vi "PathPlanner_Ctrl_LTVExecute.vi"(4 "Period":dbl=0.02, 5 "LTV_Unicycle_Ctrl_Model":T1={"Max linear ctrl effort M/S"=1.0, "Max angular ctrl effort Rad/S"=2.0, "Max Heading Meas Tol Rad"=0.2, "Max X Pos Meas Tol M"=0.0625, "Max Y Pos Meas Tol M"=0.125, "Max Linear Vel M/S"=9.0} {"Max Linear Vel M/S" format="%#_13g"; "Max Y Pos Meas Tol M" format="%#_13g"; "Max X Pos Meas Tol M" format="%#_13g"; "Max Heading Meas Tol Rad" format="%#_13g"; "Max angular ctrl effort Rad/S" format="%#_13g"; "Max linear ctrl effort M/S" format="%#_13g"}, 6 "Max Speed M/S":dbl=4.0, 7 "LTV_Unicycle_Ctrl_Tolerance":T2={"Max Heading Tolerance Rad"=1.0, "Max X Tolerance M"=2.0, "Max Y Tolerance M"=0.2} {"Max Y Tolerance M" format="%#_13g"; "Max X Tolerance M" format="%#_13g"; "Max Heading Tolerance Rad" format="%#_13g"}, 8 "Enabled":bool=TRUE, 9 "Track Width Meters":dbl=1.0, 10 "PathPlannerState":T8={"TimeSeconds"=0.0, "VelocityMPS"=0.0, "AccerationMpsSq"=0.0, "HeadingAngularVelRadPerSec"=0.0, "PositionMeters"={"X"=0.0, "Y"=0.0}, "Heading"={"VALUE"=0.0, "COS"=1.0, "SIN"=0.0}, "TargetHolonomicRotation"={"VALUE"=0.0, "COS"=1.0, "SIN"=0.0}, "CurvatureRadPerMeter"=0.0, "PathPlannerConstraints"={"MaxVelocityMps;"=0.0, "MaxAccelerationMpsSq;"=0.0, "MaxAngularVelRadPsEc;"=0.0, "MaxAngularAccRadPSecSq"=0.0, "Exists"=FALSE}, "DeltaPos"=0.0} {"TargetHolonomicRotation"."SIN" format="%13.4f"; "TargetHolonomicRotation"."COS" format="%13.4f"; "TargetHolonomicRotation"."VALUE" format="%13.4f"; "Heading"."SIN" format="%13.4f"; "Heading"."COS" format="%13.4f"; "Heading"."VALUE" format="%13.4f"; "PositionMeters"."Y" format="%14.3f"; "PositionMeters"."X" format="%14.3f"}, 11 "Current Pose SI":T4={"TRANSLATION"={"X"=0.0, "Y"=0.0}, "ROTATION"={"VALUE"=0.0, "COS"=1.0, "SIN"=0.0}} {"ROTATION"."SIN" format="%13.4f"; "ROTATION"."COS" format="%13.4f"; "ROTATION"."VALUE" format="%13.4f"; "TRANSLATION"."Y" format="%14.3f"; "TRANSLATION"."X" format="%14.3f"}) -> (0 "Position Error M":dbl, 1 "At Reference":bool, 2 "Normalized Right Wheel Dmd M/S":dbl, 3 "Normalized Left Wheel Dmd M/S":dbl)   [LabVIEW 2019, in "PathPlanner24.lvlib"]
doc: "Calculates the next output of the path following controller for differential drive robots using a LTV (linear time varying) Unicycle controller. This wraps a LTV Control function with the particulars needed to follow a PathPlanner trajectory.\n\nInputs:\n - LTV_Unicycle_Ctrl_Model - cluster - The modeling paraameters for the LTV drive controller. These are static. They should not be changed after the first call to this function.\n - UniCycle_Ctrl_Tolerance SI - pose2d - The control paraameters for the LTV drive controller. These are static. They should not be changed after the first call to this function.\n - CurrentPoseSi - pose2d - The current pose calculated by odometry or pose estimation. The pose can be absolute or relative depending on what type of trajectory is being followed.\n - PathPlannerState - cluster - The path palnner trajectory state containing the desired position and velocities of the robot.\n - TrackWidth M - doubler - The effective width of the drive track width in meters.:\n - Enabled - boolean - When TRUE, closed loop control is enabled. (Optional. Default: TRUE)\n - MaxWheelSpeed - double - The maximum speed of the drive wheels M/S.\n - Period - double - The loop period in seconds for this controller. (Optional. Default: 0.020)\n\nOutputs:\n - NormalizedLeftWheelSpeedDmd - The desired speed for the left drive wheel in SI units. The left and right speeds have been normalized so not to exceed the maximum allowed speed.\n - NormalizedRightWheelSpeedDmd - The desired speed for the right drive wheel in SI units. The left and right speeds have been normalized so not to exceed the maximum allowed speed.\n - AtReference - boolean - TRUE if the robots position is within the defined tolerance.\n - PositionError - double - Position error in SI units. How far the robot is away from the desired trajectory position."
uses:
  PathPlanner24.lvlib
  <vilib>/Rock Robotics/WPI/ThirdParty/JAS_Junk/TrajLib/TypeDef/POSE2D.ctl
  <vilib>/Rock Robotics/WPI/ThirdParty/JAS_Junk/TrajLib/TypeDef/TRANSLATION2D.ctl
  <vilib>/Rock Robotics/WPI/ThirdParty/JAS_Junk/TrajLib/TypeDef/ROTATION2D.ctl
  TypeDef/PathPlannerTrajectoryState.ctl
  TypeDef/PathPlannerPathConstraints.ctl
  <vilib>/Rock Robotics/WPI/ThirdParty/JAS_Junk/TrajLib/TypeDef/LTV_UNICYCLE_CONTROLLER.ctl
  <vilib>/Rock Robotics/WPI/ThirdParty/JAS_Junk/TrajLib/TypeDef/FUNCTION_GENERATOR_MATRIX.ctl
  <vilib>/Rock Robotics/WPI/ThirdParty/JAS_Junk/TrajLib/TypeDef/LTV_UNICYCLE_CONTROLLER_TOLERANCE.CTL
  <vilib>/Rock Robotics/WPI/ThirdParty/JAS_Junk/TrajLib/TypeDef/LTV_UNICYCLE_CONTROLLER_MODEL_PARAMS.CTL
  <vilib>/Rock Robotics/SystemInterfaces/NetworkCommunication/NetComm_UsageReport_report.vi
  <vilib>/Rock Robotics/WPI/ThirdParty/JAS_Junk/TrajLib/Pose2d_New_TRRO.vi
  <vilib>/Rock Robotics/WPI/ThirdParty/JAS_Junk/TrajLib/Util_CalcDist.vi
  <vilib>/Rock Robotics/WPI/ThirdParty/JAS_Junk/TrajLib/Globals/Util_LibraryGlobals.vi
  <vilib>/Rock Robotics/WPI/ThirdParty/JAS_Junk/TrajLib/Trajectory_Library.lvlib
panel:
  out "Error":bool
  out "out LTV_UNICYCLE_CONTROLLER":T3={"States"=0, "Inputs"=0, "PoseError"={"TRANSLATION"={"X"=0.0, "Y"=0.0}, "ROTATION"={"VALUE"=0.0, "COS"=1.0, "SIN"=0.0}}, "PoseTolerance"={"TRANSLATION"={"X"=0.0, "Y"=0.0}, "ROTATION"={"VALUE"=0.0, "COS"=1.0, "SIN"=0.0}}, "Dt"=0.02, "Enabled"=FALSE, "LQR_K_Table"={"Table Xs"=[], "Table Ys"=[], "MinX"=0.0, "MaxX"=0.0, "ItemCount"=0, "Rows"=0, "Columns"=0}} {"PoseTolerance"."ROTATION"."SIN" format="%13.4f"; "PoseTolerance"."ROTATION"."COS" format="%13.4f"; "PoseTolerance"."ROTATION"."VALUE" format="%13.4f"; "PoseTolerance"."TRANSLATION"."Y" format="%14.3f"; "PoseTolerance"."TRANSLATION"."X" format="%14.3f"; "PoseError"."ROTATION"."SIN" format="%13.4f"; "PoseError"."ROTATION"."COS" format="%13.4f"; "PoseError"."ROTATION"."VALUE" format="%13.4f"; "PoseError"."TRANSLATION"."Y" format="%14.3f"; "PoseError"."TRANSLATION"."X" format="%14.3f"}
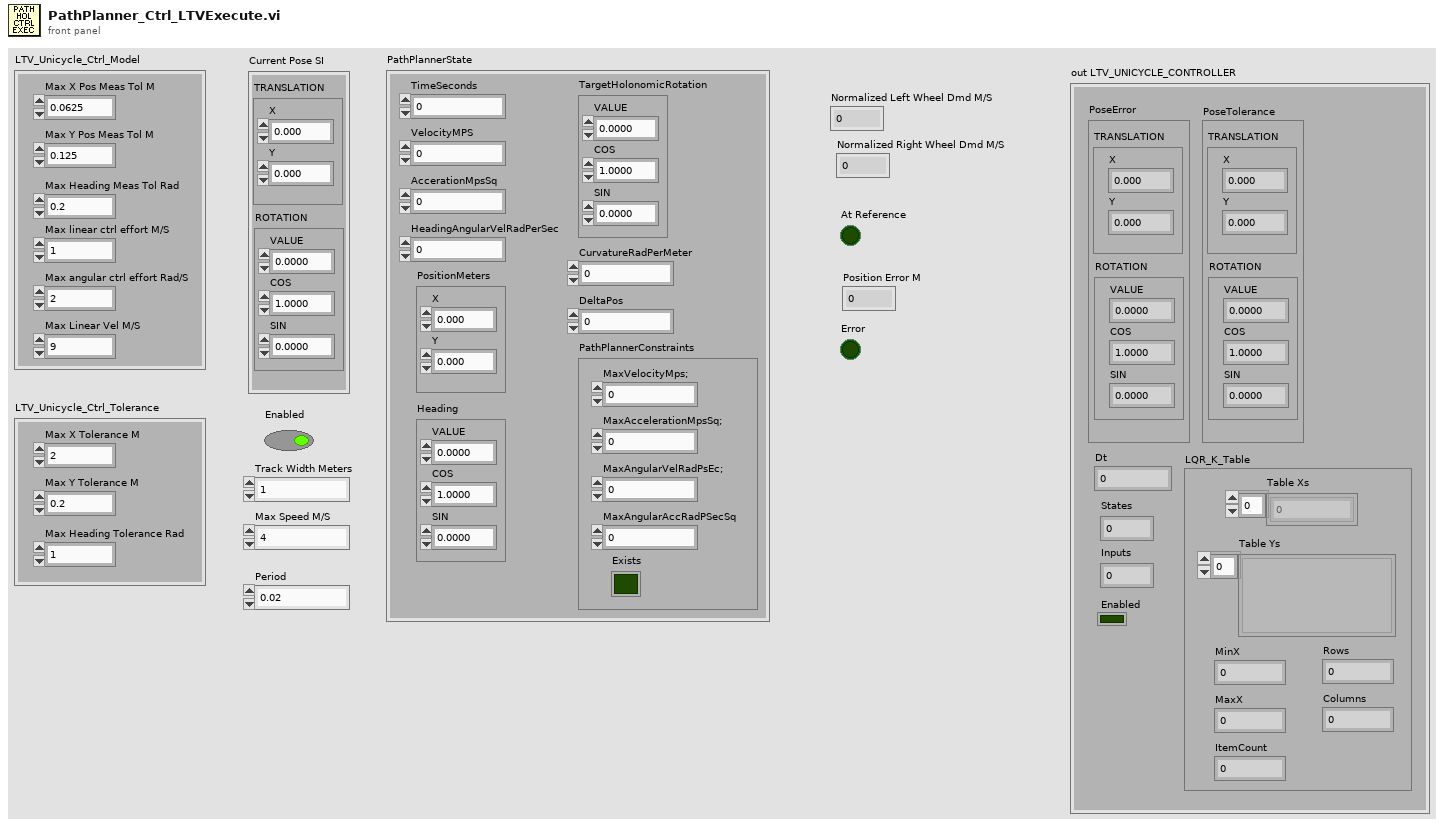
[diagram p1: front panel]
types:
  T1 = typedef "Trajectory_Library.lvlib/LTV_UNICYCLE_CONTROLLER_MODEL_PARAMS.CTL" = cluster{"Max linear ctrl effort M/S":dbl, "Max angular ctrl effort Rad/S":dbl, "Max Heading Meas Tol Rad":dbl, "Max X Pos Meas Tol M":dbl, "Max Y Pos Meas Tol M":dbl, "Max Linear Vel M/S":dbl}
  T2 = typedef "Trajectory_Library.lvlib/LTV_UNICYCLE_CONTROLLER_TOLERANCE.CTL" = cluster{"Max Heading Tolerance Rad":dbl, "Max X Tolerance M":dbl, "Max Y Tolerance M":dbl}
  T3 = typedef "Trajectory_Library.lvlib/LTV_UNICYCLE_CONTROLLER.ctl" = cluster{"States":i32, "Inputs":i32, "PoseError":T4, "PoseTolerance":T4, "Dt":dbl, "Enabled":bool, "LQR_K_Table":T7}
  T4 = typedef "Trajectory_Library.lvlib/POSE2D.ctl" = cluster{"TRANSLATION":T5, "ROTATION":T6}
  T5 = typedef "Trajectory_Library.lvlib/TRANSLATION2D.ctl" = cluster{"X":dbl, "Y":dbl}
  T6 = typedef "Trajectory_Library.lvlib/ROTATION2D.ctl" = cluster{"VALUE":dbl, "COS":dbl, "SIN":dbl}
  T7 = typedef "Trajectory_Library.lvlib/FUNCTION_GENERATOR_MATRIX.ctl" = cluster{"Table Xs":dbl[], "Table Ys":variant[], "MinX":dbl, "MaxX":dbl, "ItemCount":i32, "Rows":i32, "Columns":i32}
  T8 = typedef "PathPlanner24.lvlib/PathPlannerTrajectoryState.ctl" = cluster{"TimeSeconds":dbl, "VelocityMPS":dbl, "AccerationMpsSq":dbl, "HeadingAngularVelRadPerSec":dbl, "PositionMeters":T5, "Heading":T6, "TargetHolonomicRotation":T6, "CurvatureRadPerMeter":dbl, "PathPlannerConstraints":T9, "DeltaPos":dbl}
  T9 = typedef "PathPlanner24.lvlib/PathPlannerPathConstraints.ctl" = cluster{"MaxVelocityMps;":dbl, "MaxAccelerationMpsSq;":dbl, "MaxAngularVelRadPsEc;":dbl, "MaxAngularAccRadPSecSq":dbl, "Exists":bool}
  T10 = typedef "Trajectory_Library.lvlib/DIFF_DRIVE_KINEMATICS.ctl" = cluster{"TrackWidth_Meters":dbl}
  T11 = typedef "Trajectory_Library.lvlib/CHASSIS_SPEEDS.ctl" = cluster{"vX":dbl, "vY":dbl, "vOmega":dbl}
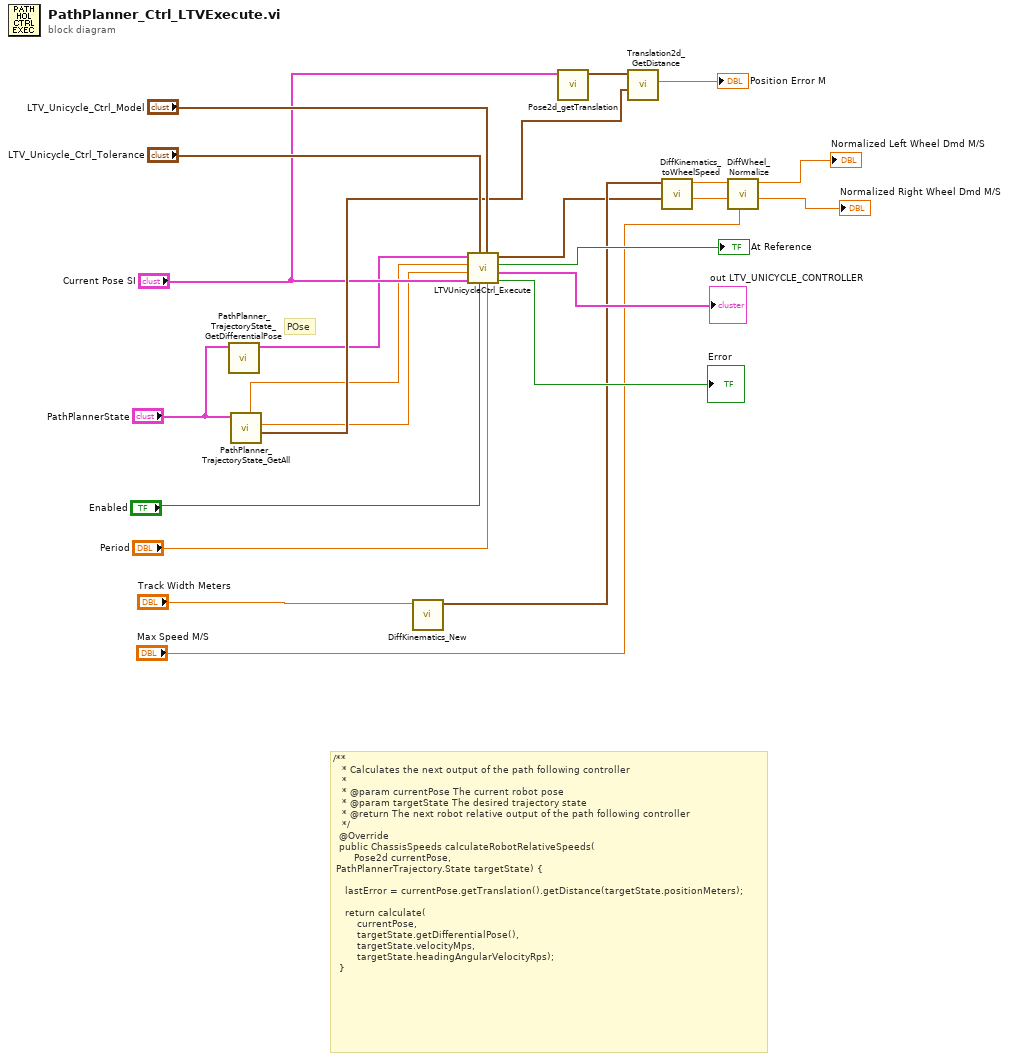
[diagram p0: block diagram]
diagram:
  # "/**\n   * Calculates the next output of the path following controller\n   *\n   * @param currentPose The current robot pose\n   * @param targetState The desired trajectory state\n   * @return The next robot relative output of the path following controller\n   */\n  @Override\n  public ChassisSpeeds calculateRobotRelativeSpeeds(\n      \tPose2d currentPose, \n\tPathPlannerTrajectory.State targetState) {\n\n    lastError = currentPose.getTranslation().getDistance(targetState.positionMeters);\n\n    return calculate(\n        currentPose,\n        targetState.getDifferentialPose(),\n        targetState.velocityMps,\n        targetState.headingAngularVelocityRps);\n  }"
  # "POse"
  n1 = call "PathPlanner_TrajectoryState_GetDifferentialPose.vi"("PathPlannerState"="PathPlannerState") -> ("DifferentialPose"=w11:T4)  [unwired: 10 in]
  n2 = call "PathPlanner_TrajectoryState_GetAll.vi"("PathPlannerState"="PathPlannerState") -> ("PositionMeters"=w15:T5, "HeadingAngularVelRadPerSec"=w9:dbl, "VelocityMPS"=w10:dbl)  [unwired: 1 in, 7 out]
  n3 = call <vilib>:"DiffKinematics_New.vi"("TrackWidth_Meters"="Track Width Meters") -> ("DIFF_DRIVE_KINEMATICS"=w5:T10)  [unwired: 10 in]
  n4 = call <vilib>:"LTVUnicycleCtrl_Execute.vi"("dT Sec"="Period", "LTV_Unicycle_Ctrl_Model"="LTV_Unicycle_Ctrl_Model", "Enabled"="Enabled", "LTV_Unicycle_Ctrl_Tolerance"="LTV_Unicycle_Ctrl_Tolerance", "CurrentPose"="Current Pose SI", "RefAngularVelocity"=w9, "RefLinearVelocity"=w10, "RefPose"=w11) -> ("Error"=→"Error":bool, "out LTV_UNICYCLE_CONTROLLER"=→"out LTV_UNICYCLE_CONTROLLER":T3, "At Reference"=→"At Reference":bool, "ChassisSpeeds"=w4:T11)
  n5 = call <vilib>:"Pose2d_getTranslation.vi"("in POSE"="Current Pose SI") -> ("outTRANSLATION"=w16:T5)  [unwired: 10 in]
  n6 = call <vilib>:"Translation2d_GetDistance.vi"("other Translation"=w15, "In Translation"=w16) -> ("Distance"=→"Position Error M":dbl)  [unwired: 9 in]
  n7 = call <vilib>:"DiffKinematics_toWheelSpeed.vi"("CHASSIS Speed"=w4, "DIFF_DRIVE_KINEMATICS"=w5) -> ("RightVelocity"=w7:dbl, "LeftVelocity"=w8:dbl)  [unwired: 8 in]
  n8 = call <vilib>:"DiffWheel_Normalize.vi"("Max Speed"="Max Speed M/S", "Right Wheel Demand"=w7, "Left Wheel Demand"=w8) -> ("Normalized Right Wheel Demand"=→"Normalized Right Wheel Dmd M/S":dbl, "Normalized Left Wheel Demand"=→"Normalized Left Wheel Dmd M/S":dbl)  [unwired: 7 in]
